vi "ButtonGroupEnum Example.vi"() -> ()   [LabVIEW 2017, in "ButtonGroupEnum.lvlib"]
doc: "Example VI showing how a group of boolean buttons is read as and written from an enum, using ButtonGroupEnum to Enum.vim and Set ButtonGroupEnum Value.vim inside an event loop."
uses:
  ButtonGroupEnum.lvlib
  e4533dfa-7e56-4b80-ad66-7e72ac4606b5.vi
  ca3ba9a0-c577-455f-81d4-0b62f7062e71.vi
  f68442da-1146-4dbf-ba63-0d1de55603c9.vi
  _support/_Set ButtonGroupEnum Value.vi
  _support/_ButtonGroupEnum to Num.vi
  Set ButtonGroupEnum By Ref.vi
panel:
  in  "Type":enum16{"Sine", "Triangle", "Square", "DC"}(ring)
  in  "DC":bool
  in  "Triangle":bool caption="三角波"
  in  "Sine":bool caption="正弦波"
  in  "Square":bool caption="方波"
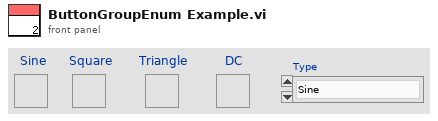
[diagram p1: front panel]
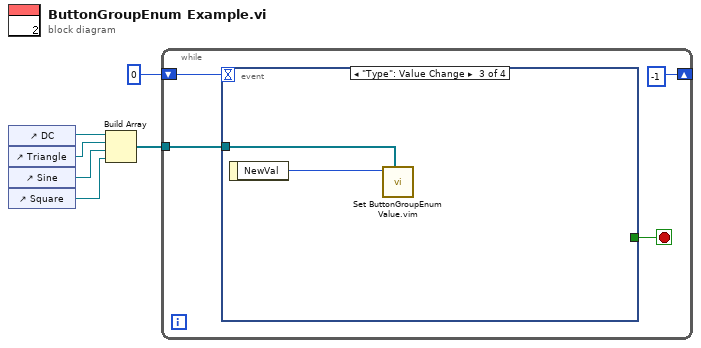
[diagram p0: block diagram]
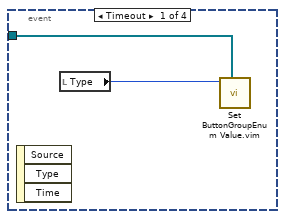
[diagram p2: hidden frame]
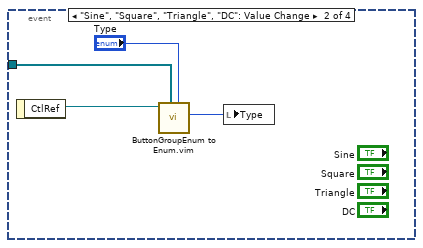
[diagram p3: hidden frame]
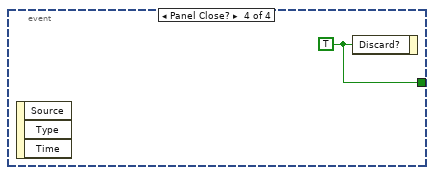
[diagram p4: hidden frame]
diagram:
  n1 = control-ref of="DC"() -> (w5:refnum<vi>)
  n2 = control-ref of="Triangle"() -> (w4:refnum<vi>)
  n3 = control-ref of="Sine"() -> (w3:refnum<vi>)
  n4 = control-ref of="Square"() -> (w2:refnum<vi>)
  n5 = Build Array(w5, w4, w3, w2) -> (w1:refnum<vi>[])
  n6 = while {
    shift-right: [-1] -> _
    shift-left: 0 -> [w9]
    tunnel: w1 -> [w7]
    stop <- w10 stop-if-true
    n7 = event shown="[2] \"Type\": Value Change" {
      selector: _ -> [_ _ _ _]
      dyn-events: _ -> [_ _ _ _]
      timeout: w9 -> [_ _ _ _]
      tunnel: [_ _ _ w19] -> w10
      tunnel: w7 -> [w12 w16 w18 _]
      event Timeout {
        n8 = event-data() -> ()  [unwired: 1 in, 3 out]
        n9 = local read "Type"() -> (w11:enum16{"Sine", "Triangle", "Square", "DC"})
        n10 = call "Set ButtonGroupEnum Value.vim"("ModeBtnRefs"=w12, "Enum"=w11) -> ()  [unwired: 9 in, 1 out]
      }
      event "Sine", "Square", "Triangle", "DC": Value Change {
        n11 = event-data() -> ("CtlRef"=w15:refnum<vi>)  [unwired: 1 in]
        n12 = call "ButtonGroupEnum to Enum.vim"("Enum"="Type", "ModeBtnRefs"=w16, "CtlRef"=w15) -> ("Enum (dup)"=w14:enum16{"Sine", "Triangle", "Square", "DC"})  [unwired: 6 in, 2 out]
        n13 = local write "Type"(w14) -> ()
      }
      event "Type": Value Change {
        n14 = event-data() -> ("NewVal"=w17:enum16{"Sine", "Triangle", "Square", "DC"})  [unwired: 1 in]
        n15 = call "Set ButtonGroupEnum Value.vim"("ModeBtnRefs"=w18, "Enum"=w17) -> ()  [unwired: 9 in, 1 out]
      }
      event Panel Close? {
        w19 = TRUE ("Discard?")
        n16 = event-data() -> ()  [unwired: 1 in, 3 out]
        n17 = event-data("Discard?"=w19) -> ()  [unwired: 1 in, 1 out]
      }
    }
  }
